vi "niFPGA Memory Element_m.vi"   [LabVIEW 2017]
doc: "Stores the input value and returns it on the next call. The data type you wire to <B>input</B> determines the <B>output</B> data type."
uses:
  <vilib>/rvi/Analysis/common/FxpNativeNode/niFpgaFxpNative.xnode
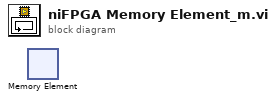
[diagram p0: block diagram]
diagram:
  n1 = xnode "Memory Element"() -> ()  [unwired: 3 in, 1 out]
